vi "Interpret WiFi101 status.vi"(1 "WiFi Status\nCode":u8) -> (4 "Connected to network?":bool, 5 "Feather Wifi Status":T1 items=["No module"=255, "Idle"=0, "No SSID"=1, "Scan completed"=2, "Connected"=3, "Connection failed"=4, "Connection lost"=5, "Disconnected"=6, "AP listening"=7, "AP connected"=8, "AP failed"=9, "Provisioning"=10, "Provisioning failed"=11])   [LabVIEW 2019, in "LINXx.lvlib"]
doc: "Interpret WiFI101 connection status"
uses:
  LINXx.lvlib
  Private/WiFi101 Status.ctl
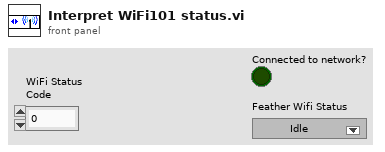
[diagram p1: front panel]
types:
  T1 = typedef "LINXx.lvlib/WiFi101 Status.ctl" = u8
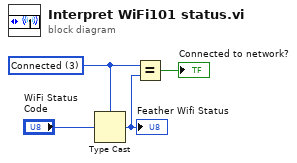
[diagram p0: block diagram]
diagram:
  w3 = T1 3 items=["No module"=255, "Idle"=0, "No SSID"=1, "Scan completed"=2, "Connected"=3, "Connection failed"=4, "Connection lost"=5, "Disconnected"=6, "AP listening"=7, "AP connected"=8, "AP failed"=9, "Provisioning"=10, "Provisioning failed"=11] ("Ring")
  n1 = Type Cast(type=w3, x="WiFi Status\nCode") -> (*(type *) &x=w2:T1)
  "Feather Wifi Status" <- w2
  n2 = Equal?(x=w3, y=w2) -> (x = y?=→"Connected to network?":bool)
